vi "000_Control Value.vi"(9 "Value In":variant, 10 "Value String In":string, 11 "Class Name":string) -> (1 "Value String Out":string, 2 "Value Out":variant)   [LabVIEW 2020]
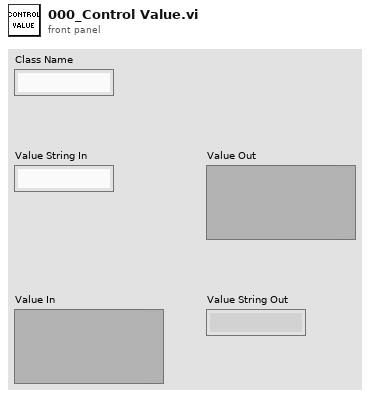
[diagram p1: front panel]
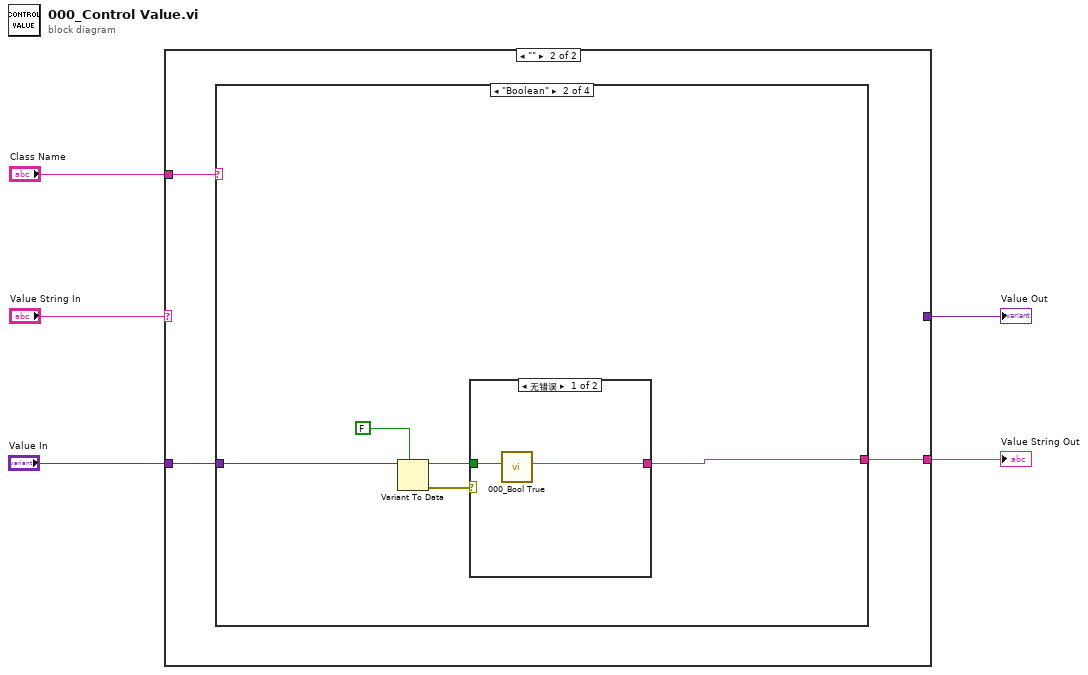
[diagram p0: block diagram]
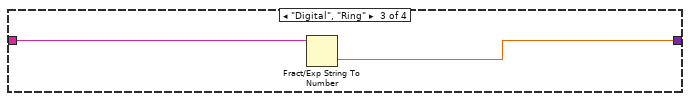
[diagram p4: hidden frame]
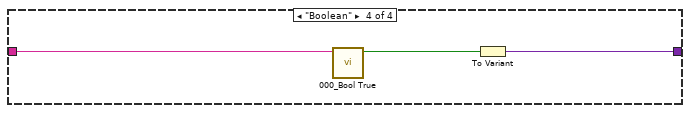
[diagram p5: hidden frame]
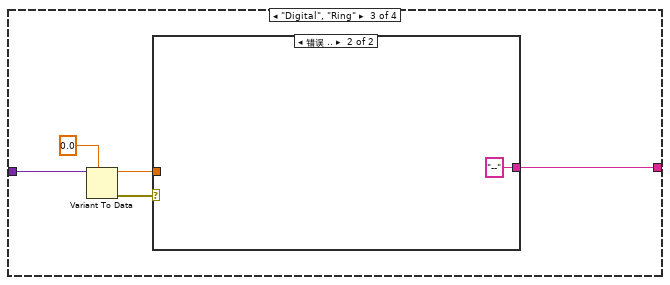
[diagram p8: hidden frame]
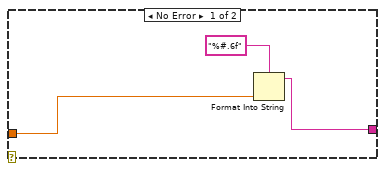
[diagram p9: hidden frame]
diagram:
  n1 = case shown="\"\"" "Value String In" {
    selector: "Value String In" -> [w7 _]
    tunnel: "Value In" -> [w8 w17]
    tunnel: "Class Name" -> [w9 w18]
    tunnel: [w6 _] -> w2
    tunnel: [_ w16] -> w1
    frame "eee", Default {
      n2 = case shown="\"String\"" w9 {
        tunnel: w8 -> [_ _ _ _]
        tunnel: w7 -> [_ w10 w12 w15]
        tunnel: [_ w10 w11 w13] -> w6
        frame "eee", Default {
        }
        frame "String" {
        }
        frame "Digital", "Ring" {
          n3 = Fract/Exp String To Number(string=w12) -> (number=w11:dbl)  [unwired: 3 in, 1 out]
        }
        frame "Boolean" {
          n4 = call "000_Bool True.vi"("Bool String"=w15) -> ("True"=w14:bool)  [unwired: 8 in, 2 out]
          n5 = To Variant(anything=w14) -> (Variant=w13:variant)
        }
      }
    }
    frame "" {
      n6 = case shown="\"Boolean\"" w18 {
        tunnel: w17 -> [_ w23 w30 _]
        tunnel: [_ w20 w27 _] -> w16
        frame "eee", Default {
        }
        frame "Boolean" {
          n7 = Variant To Data(type=FALSE, Variant=w23) -> (data=w21:bool, error out=w19:errorcluster)  [unwired: 1 in]
          n8 = case shown="无错误" w19 {
            tunnel: w21 -> [w25 _]
            tunnel: [w24 _] -> w20
            frame No Error {
              n9 = call "000_Bool True.vi"("Value"=w25) -> ("String Out"=w24:string)  [unwired: 8 in, 2 out]
            }
            frame Error {
            }
          }
        }
        frame "Digital", "Ring" {
          n10 = Variant To Data(type=0.0, Variant=w30) -> (data=w28:dbl, error out=w26:errorcluster)  [unwired: 1 in]
          n11 = case shown="错误 .." w26 {
            tunnel: w28 -> [w32 _]
            tunnel: [w31 "--"] -> w27
            frame No Error {
              n12 = Format Into String(format string="%#.6f" ("格式字符串"), w32) -> (resulting string=w31:string)  [unwired: 2 in, 1 out]
            }
            frame Error {
            }
          }
        }
        frame "String" {
        }
      }
    }
  }
  "Value String Out" <- w1
  "Value Out" <- w2
